vi "paying.vi"(0 "Total Amount(In)":i32) -> (1 "Boolean":bool, 2 "Next state":T1(ring), 3 "Leave":bool)   [LabVIEW 2014]
panel:
  out "Boolean 2":bool
  out "Total Amount":i32
  out "Deposition":i32
  in  "Cluster":T2
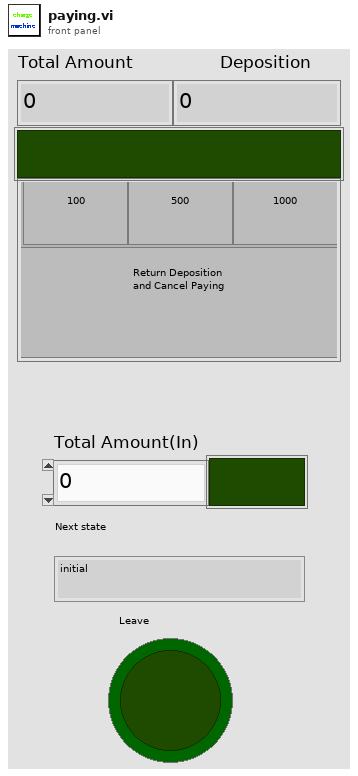
[diagram p1: front panel]
types:
  T1 = enum16{"initial", "start", "member?", "register?", "member login", "member register", "choose movie", "how many seat?", "check", "end"}
  T2 = cluster{"OK Button":bool, "OK Button 2":bool, "OK Button 3":bool, "OK Button 5":bool}
  T3 = enum16{"Wait Button Pressed", "100 coin added", "500 coin added", "1000 coin added", "dispensing event", "deposition enough?", "End", "Cancel"}
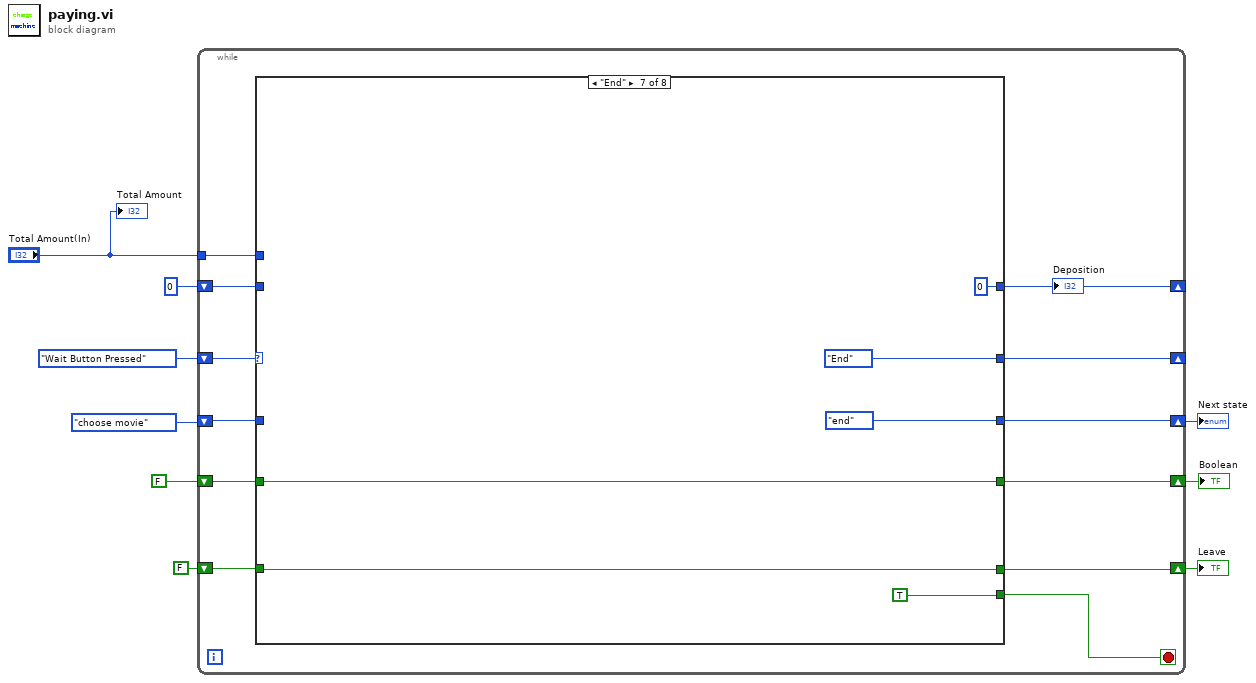
[diagram p0: block diagram]
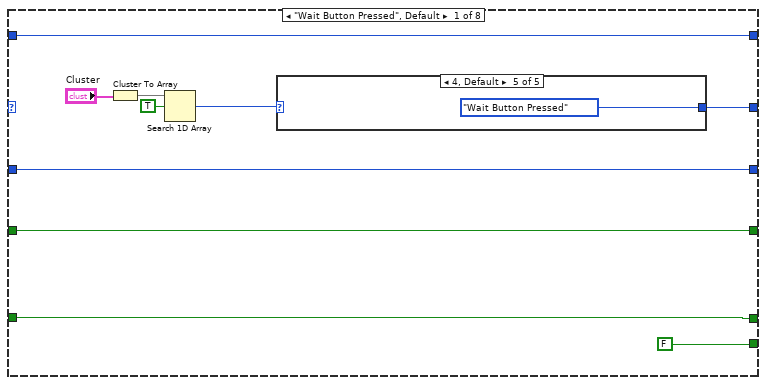
[diagram p2: hidden frame]
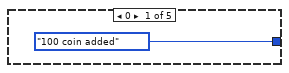
[diagram p3: hidden frame]
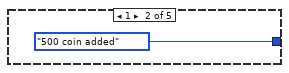
[diagram p4: hidden frame]
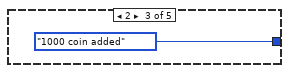
[diagram p5: hidden frame]
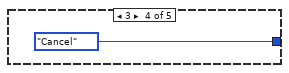
[diagram p6: hidden frame]
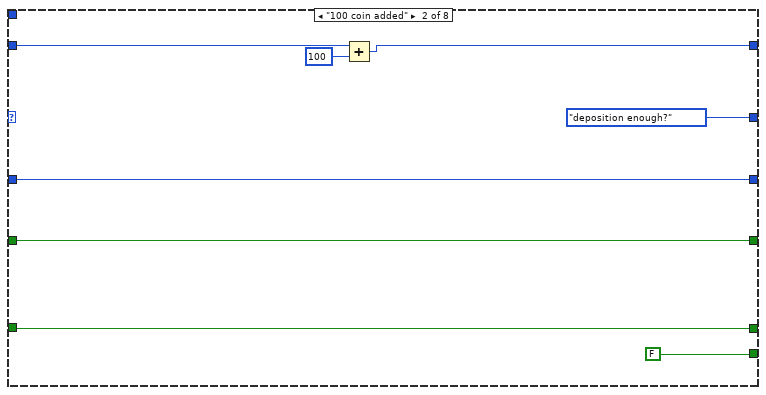
[diagram p7: hidden frame]
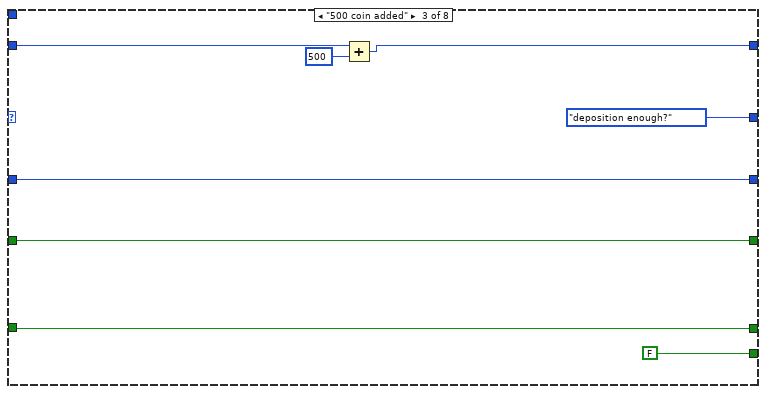
[diagram p8: hidden frame]
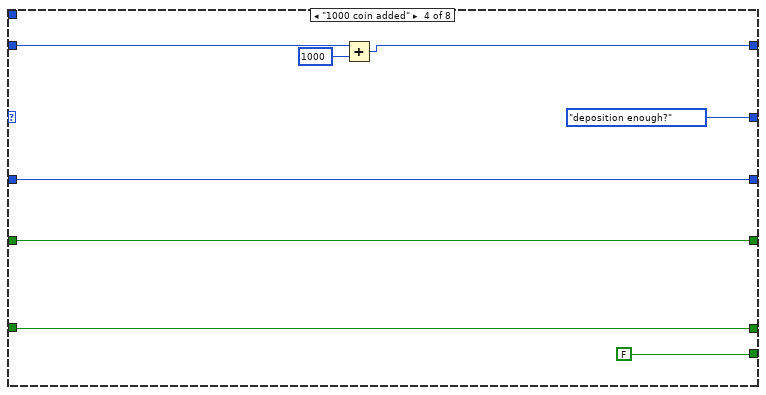
[diagram p9: hidden frame]
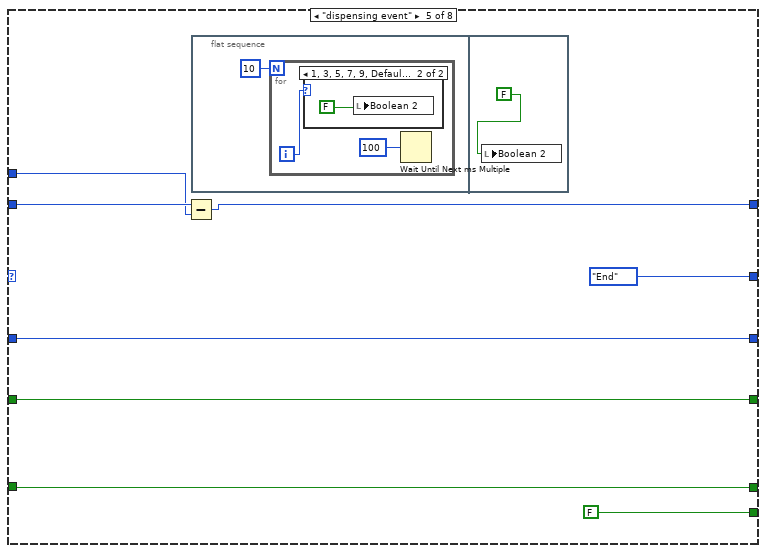
[diagram p10: hidden frame]
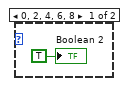
[diagram p11: hidden frame]
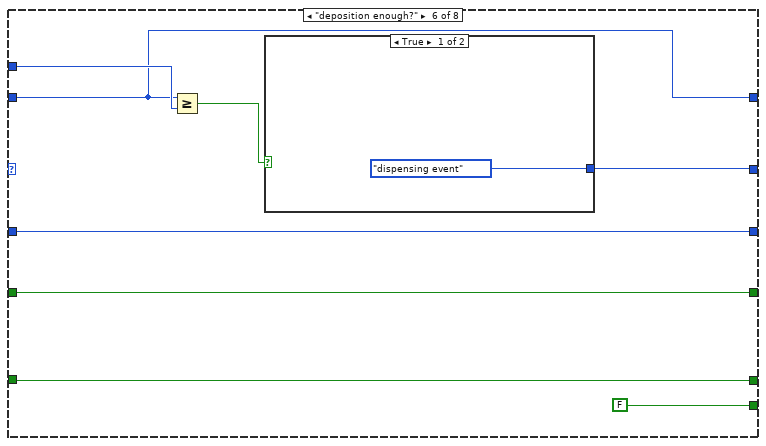
[diagram p12: hidden frame]
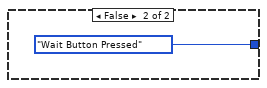
[diagram p13: hidden frame]
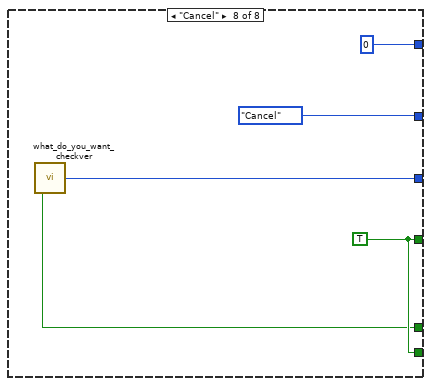
[diagram p14: hidden frame]
diagram:
  n1 = while {
    shift-right: [w20] -> _
    shift-left: T3."Wait Button Pressed" -> [w21]
    shift-right: [w18] -> _
    shift-left: 0 -> [w19]
    tunnel: "Total Amount(In)" -> [w17]
    shift-right: [w15] -> w5
    shift-left: FALSE -> [w16]
    shift-right: [w14] -> w4
    shift-left: T1."choose movie" -> [w13]
    shift-right: [w11] -> w2
    shift-left: FALSE ("Leave") -> [w10]
    stop <- w12 stop-if-true
    n2 = case shown="\"End\"" w21 {
      tunnel: [w27 T3."deposition enough?" T3."deposition enough?" T3."deposition enough?" T3."End" w80 T3."End" T3."Cancel"] -> w20
      tunnel: w19 -> [w26 w44 w52 w60 w68 w79 _ _]
      tunnel: [w26 w42 w50 w58 w66 w79 0 0] -> w18
      tunnel: w17 -> [_ _ _ _ w67 w82 _ _]
      tunnel: w16 -> [w25 w40 w48 w56 w64 w78 w88 _]
      tunnel: [w25 w40 w48 w56 w64 w78 w88 w92] -> w15
      tunnel: [w24 w39 w47 w55 w63 w77 T1."end" w93] -> w14
      tunnel: w13 -> [w24 w39 w47 w55 w63 w77 _ _]
      tunnel: [FALSE FALSE FALSE FALSE FALSE FALSE TRUE w92] -> w12
      tunnel: [w22 w37 w45 w53 w61 w75 w85 w91] -> w11
      tunnel: w10 -> [w22 w37 w45 w53 w61 w75 w85 _]
      frame "Wait Button Pressed", Default {
        n3 = Cluster To Array(cluster="Cluster") -> (array=w30:bool[])
        n4 = Search 1D Array(1D array=w30, element=TRUE) -> (index of element=w28:i32)  [unwired: 1 in]
        n5 = case shown="4, Default" w28 {
          tunnel: [T3."100 coin added" T3."500 coin added" T3."1000 coin added" T3."Cancel" T3."Wait Button Pressed"] -> w27
          frame 0 {
          }
          frame 1 {
          }
          frame 2 {
          }
          frame 3 {
          }
          frame 4, Default {
          }
        }
      }
      frame "100 coin added" {
        n6 = Add(x=w44, y=100) -> (x+y=w42:i32)
      }
      frame "500 coin added" {
        n7 = Add(x=w52, y=500) -> (x+y=w50:i32)
      }
      frame "1000 coin added" {
        n8 = Add(x=w60, y=1000) -> (x+y=w58:i32)
      }
      frame "dispensing event" {
        n9 = Subtract(x=w68, y=w67) -> (x-y=w66:i32)
        n10 = flat-sequence {
          frame #0 {
            n11 = for {
              N: 10 -> [_]
              i -> [w70]
              n12 = case shown="1, 3, 5, 7, 9, Default" w70 {
                frame 0, 2, 4, 6, 8 {
                  "Boolean 2" <- TRUE ("Boolean")
                }
                frame 1, 3, 5, 7, 9, Default {
                  n13 = local write "Boolean 2"(FALSE ("Boolean")) -> ()
                }
              }
              n14 = Wait Until Next ms Multiple(millisecond multiple=u32 100) -> ()  [unwired: 1 out]
            }
          }
          frame #1 {
            n15 = local write "Boolean 2"(FALSE) -> ()
          }
        }
      }
      frame "deposition enough?" {
        n16 = Greater Or Equal?(x=w79, y=w82) -> (x >= y?=w81:bool)
        n17 = case shown="True" w81 {
          tunnel: [T3."dispensing event" T3."Wait Button Pressed"] -> w80
          frame True {
          }
          frame False {
          }
        }
      }
      frame "End" {
      }
      frame "Cancel" {
        w92 = TRUE
        n18 = call "what_do_you_want_checkver.vi"() -> ("Next state"=w93:T1, "Leave"=w91:bool)
      }
    }
    "Deposition" <- w18
  }
  "Boolean" <- w5
  "Next state" <- w4
  "Leave" <- w2
  "Total Amount" <- "Total Amount(In)"
